vi "Send Data to Dashboard.vi"() -> ()   [LabVIEW 2013]
uses:
  <vilib>/Rock Robotics/WPI/DriverStation/WPI_DriverStationRobotMode2.ctl
  Globals/Useful Values.vi
  Globals/Enables.vi
  <vilib>/Utility/file.llb/Read From Spreadsheet File (I64).vi
  Globals/Data for Dashboard.vi
  Robot Global Data.vi
panel:
  out "Boolean array":bool[](array[boolean])
  out "data out":string
  out "String to Send":string
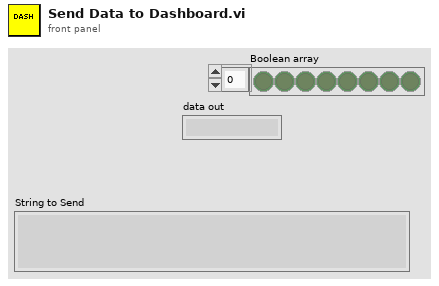
[diagram p1: front panel]
types:
  T1 = typedef "WPI_DriverStationRobotMode2.ctl" = enum16{"Autonomous Disabled", "Autonomous Enabled", "Teleop Disabled", "Teleop Enabled", "Timeout", "Finish", "Test Disabled", "Test Enabled"}
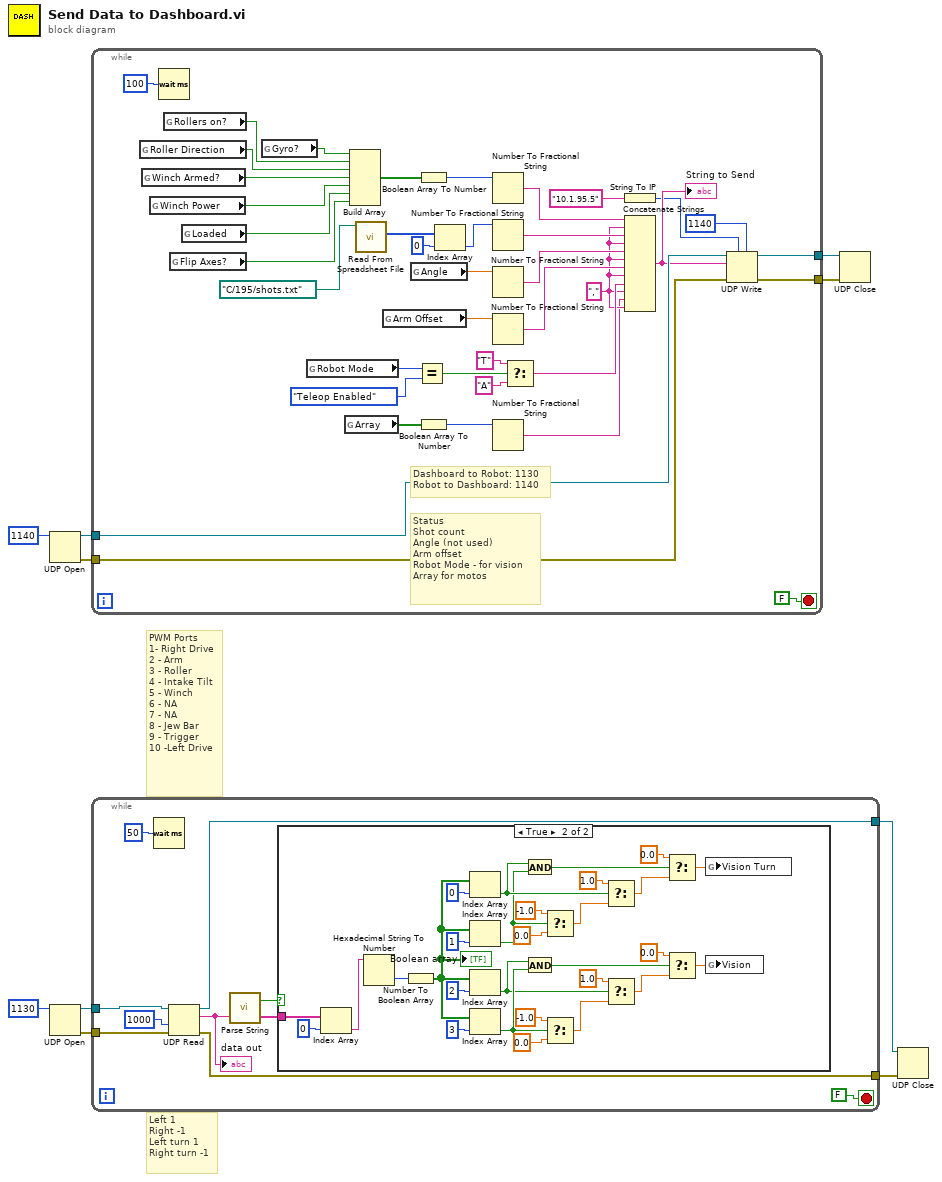
[diagram p0: block diagram]
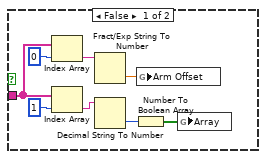
[diagram p2: hidden frame]
diagram:
  # "Left 1\nRight -1\nLeft turn 1\nRight turn -1"
  # "PWM Ports\n1- Right Drive\n2 - Arm\n3 - Roller\n4 - Intake Tilt \n5 - Winch\n6 - NA \n7 - NA\n8 - Jew Bar\n9 - Trigger\n10 -Left Drive"
  n1 = UDP Open(11:u16 1140 ("port")) -> (port=w10:refnum<k16>, 0:w9:errorcluster)  [unwired: 4 in, 1 out]
  n2 = UDP Open(11:u16 1130 ("port")) -> (port=w4:refnum<k16>, 0:w3:errorcluster)  [unwired: 4 in, 1 out]
  n3 = while {
    tunnel: w10 -> [w36]
    tunnel: w9 -> [w35]
    tunnel: [w34] -> w8
    tunnel: [w33] -> w7
    stop <- FALSE stop-if-true
    w14 = ","
    # "Status\nShot count\nAngle (not used)\nArm offset\nRobot Mode - for vision\nArray for motos"
    # "Dashboard to Robot: 1130\nRobot to Dashboard: 1140"
    n4 = global read "Data for Dashboard.vi" "Roller Direction"() -> (w45:bool)
    n5 = global read "Data for Dashboard.vi" "Winch Armed?"() -> (w44:bool)
    n6 = global read "Data for Dashboard.vi" "Winch Power"() -> (w43:bool)
    n7 = Wait (ms)(milliseconds to wait=u32 100) -> ()  [unwired: 1 out]
    n8 = global read "Data for Dashboard.vi" "Rollers on?"() -> (w46:bool)
    n9 = global read "Data for Dashboard.vi" "Flip Axes?"() -> (w41:bool)
    n10 = global read "Data for Dashboard.vi" "Loaded"() -> (w42:bool)
    n11 = global read "Data for Dashboard.vi" "Gyro?"() -> (w47:bool)
    n12 = global read "Robot Global Data.vi" "Robot Mode"() -> (w20:T1)
    n13 = global read "Enables.vi" "Array"() -> (w13:bool[])
    n14 = Build Array(w47, w46, w45, w44, w43, w42, w41) -> (w40:bool[])
    n15 = call-poly <vilib>:"Read From Spreadsheet File.vi"("file path (dialog if empty)"=path "C:/195/shots.txt" ("path")) -> ("first row"=w39:i64[])  [unwired: 6 in, 4 out]
    n16 = global read "Useful Values.vi" "Arm Offset"() -> (w22:dbl)
    n17 = global read "Data for Dashboard.vi" "Angle"() -> (w23:dbl)
    n18 = Equal?(x=w20, y=WPI_DriverStationRobotMode2."Teleop Enabled") -> (x = y?=w18:bool)
    n19 = Boolean Array To Number(Boolean array=w40) -> (number=w30:u32)
    n20 = Boolean Array To Number(Boolean array=w13) -> (number=w12:u32)
    n21 = Index Array(array=w39, index=0) -> (element=w31:i64)
    n22 = Number To Fractional String(number=w30) -> (F-format string=w29:string)  [unwired: 3 in]
    n23 = Number To Fractional String(number=w31) -> (F-format string=w28:string)  [unwired: 3 in]
    n24 = Number To Fractional String(number=w23) -> (F-format string=w27:string)  [unwired: 3 in]
    n25 = Number To Fractional String(number=w22) -> (F-format string=w21:string)  [unwired: 3 in]
    n26 = Number To Fractional String(number=w12) -> (F-format string=w11:string)  [unwired: 3 in]
    n27 = Select(t="T", s=w18, f="A") -> (s? t:f=w15:string)
    n28 = String To IP(1:"10.1.95.5" ("name")) -> (0:w25:u32)
    n29 = Concatenate Strings(w29, w14, w28, w14, w27, w14, w21, w14, w15, w14, w11, w14) -> (w26:string)
    "String to Send" <- w26
    n30 = UDP Write(address=w25, port or service name=u16 1140, connection ID=w36, data in=w26, 8:w35) -> (error out=w34:errorcluster, 3:w33:refnum<k16>)  [unwired: 1 in]
  }
  n31 = while {
    tunnel: w4 -> [w59]
    tunnel: w3 -> [w58]
    tunnel: [w55] -> w2
    tunnel: [w57] -> w1
    stop <- FALSE stop-if-true
    n32 = Wait (ms)(milliseconds to wait=u32 50) -> ()  [unwired: 1 out]
    n33 = UDP Read(connection ID=w59, timeout ms (25000)=1000, 8:w58) -> (data out=w53:string, error out=w55:errorcluster, 3:w57:refnum<k16>)  [unwired: 3 out]
    "data out" <- w53
    n34 = call "Parse String.vi"("String In"=w53) -> ("Array Out"=w52:string[], "Source"=w50:bool)  [unwired: 1 in]
    n35 = case shown="True" w50 {
      tunnel: w52 -> [w60 w96]
      frame False {
        n36 = Index Array(array=w60, index=0) -> (element=w65:string)
        n37 = Index Array(array=w60, index=1) -> (element=w63:string)
        n38 = Fract/Exp String To Number(string=w65) -> (number=w67:dbl)  [unwired: 3 in, 1 out]
        n39 = Decimal String To Number(string=w63) -> (number=w62:i32)  [unwired: 2 in, 1 out]
        n40 = Number To Boolean Array(number=w62) -> (Boolean array=w61:bool[])
        n41 = global write "Useful Values.vi" "Arm Offset"(w67) -> ()
        n42 = global write "Enables.vi" "Array"(w61) -> ()
      }
      frame True {
        n43 = Index Array(array=w96, index=0) -> (element=w69:string)
        n44 = Hexadecimal String To Number(string=w69) -> (number=w68:u32)  [unwired: 2 in, 1 out]
        n45 = Number To Boolean Array(number=w68) -> (Boolean array=w74:bool[])
        "Boolean array" <- w74
        n46 = Index Array(array=w74, index=0) -> (element=w88:bool)
        n47 = Index Array(array=w74, index=1) -> (element=w87:bool)
        n48 = Index Array(array=w74, index=2) -> (element=w72:bool)
        n49 = Index Array(array=w74, index=3) -> (element=w73:bool)
        n50 = And(x=w88, y=w87) -> (x .and. y?=w86:bool)
        n51 = And(x=w72, y=w73) -> (x .and. y?=w79:bool)
        n52 = Select(t=-1.0, s=w87, f=0.0) -> (s? t:f=w89:dbl)
        n53 = Select(t=-1.0, s=w73, f=0.0) -> (s? t:f=w78:dbl)
        n54 = Select(t=1.0, s=w88, f=w89) -> (s? t:f=w84:dbl)
        n55 = Select(t=1.0, s=w72, f=w78) -> (s? t:f=w81:dbl)
        n56 = Select(t=0.0, s=w86, f=w84) -> (s? t:f=w71:dbl)
        n57 = Select(t=0.0, s=w79, f=w81) -> (s? t:f=w70:dbl)
        n58 = global write "Useful Values.vi" "Vision Turn"(w71) -> ()
        n59 = global write "Useful Values.vi" "Vision"(w70) -> ()
      }
    }
  }
  n60 = UDP Close(connection ID=w7, 8:w8) -> ()  [unwired: 2 out]
  n61 = UDP Close(connection ID=w1, 8:w2) -> ()  [unwired: 2 out]
